vi "Main.vi"(8 "error in":errorcluster, 10 "Sequence Context":refnum<k7>, 11 "PostUUT":refnum<class "PostUUT.lvclass">) -> (0 "error out":errorcluster, 3 "PostUUT":refnum<class "PostUUT.lvclass">)   [LabVIEW 2019, in "Sequence Main.lvlib" / "PostUUT.lvclass"]
uses:
  PostUUT.lvclass
  C:/Workspace/gip-fct/Sequence/CodeModules/PreTestPost Launcher/Abstract UUT/Abstract UUT.lvclass
  PostUUT.lvclass/PostUUT.ctl
  Abstract UUT/Abstract UUT.lvclass
panel:
  out "MssgText":string
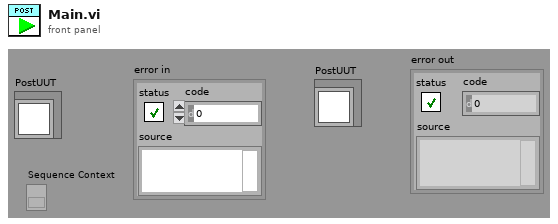
[diagram p1: front panel]
types:
  T1 = typedef "TestStand - Status Monitor.ctl" = cluster{"Sequence Context":refnum<k7>, "Execution":refnum<k7>, "Termination Monitor":refnum<k7>}
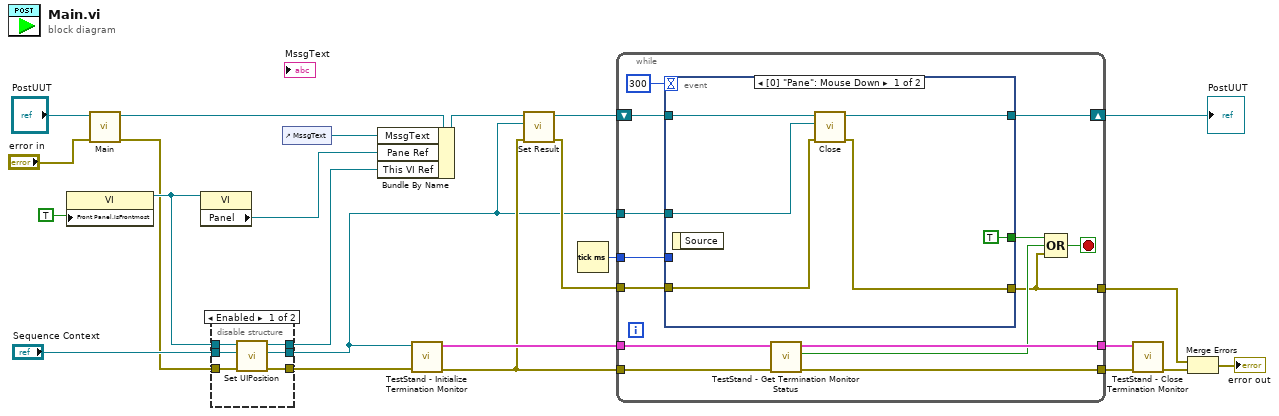
[diagram p0: block diagram]
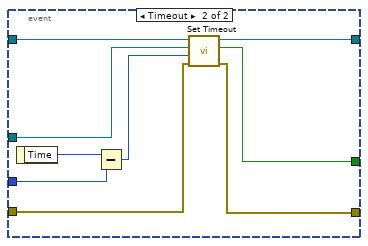
[diagram p3: hidden frame]
diagram:
  n1 = property class="VI"("Front Panel.IsFrontmost"=TRUE ("Front Panel Window:Is Frontmost")) -> (reference out=w15:refnum<vi>)  [unwired: 2 in, 1 out]
  n2 = call-parent "Main.vi"("error in"="error in", "OPC UA In"="PostUUT") -> ("error out"=w6:errorcluster, "OPC UA Out"=w7:refnum<class "PostUUT.lvclass">)  [unwired: 8 in]
  n3 = property class="VI"(reference=w15) -> ("Panel"=w23:refnum<vi>)  [unwired: 1 in, 2 out]
  n4 = disable-structure shown="Enabled" {
    disable-tunnel: [w30 w31] -> w17
    disable-tunnel: "Sequence Context" -> [w26 w32]
    disable-tunnel: w15 -> [w29 w33]
    disable-tunnel: [w28 w33] -> w14
    disable-tunnel: [w25 w32] -> w1
    disable-tunnel: w6 -> [w27 w31]
    frame Enabled {
      n5 = call "Set UIPosition.vi"("error in"=w27, "Sequence Context In"=w26, "VI Ref"=w29) -> ("error out"=w30:errorcluster, "Sequence Context out"=w25:refnum<k7>, "VI Ref out"=w28:refnum<vi>)  [unwired: 6 in]
    }
    frame Disabled {
    }
  }
  n6 = control-ref of="MssgText"() -> (w8:refnum<vi>)
  n7 = Bundle By Name(cluster=w7, "MssgText"=w8, "Pane Ref"=w23, "This VI Ref"=w14) -> (w5:refnum<class "PostUUT.lvclass">)
  n8 = call <vilib>:"TestStand - Initialize Termination Monitor.vi"("error in (no error)"=w17, "Sequence Context In"=w1) -> ("error out"=w3:errorcluster, "Status Monitor Out"=w22:T1)  [unwired: 8 in]
  n9 = call "Set Result.vi"("error in (no error)"=w3, "Sequence Context"=w1, "PostUUT in"=w5) -> ("error out"=w2:errorcluster, "PostUUT out"=w4:refnum<class "PostUUT.lvclass">)  [unwired: 7 in]
  n10 = Tick Count (ms)() -> (millisecond timer value=w11:u32)
  n11 = while {
    tunnel: w3 -> [w45]
    tunnel: w22 -> [w44]
    tunnel: [w38] -> w21
    tunnel: [w42] -> w20
    tunnel: w2 -> [w37]
    tunnel: [w36] -> w12
    tunnel: w11 -> [w35]
    shift-right: [w41] -> w9
    shift-left: w4 -> [w47]
    tunnel: w1 -> [w34]
    stop <- w43 stop-if-true
    n12 = event shown="[0] \"Pane\": Mouse Down" {
      selector: _ -> [_ _]
      dyn-events: _ -> [_ _]
      timeout: 300 -> [_ _]
      tunnel: w47 -> [w52 w60]
      tunnel: [w51 w59] -> w41
      tunnel: [TRUE ("Timeout") w56] -> w39
      tunnel: w37 -> [w50 w58]
      tunnel: [w49 w57] -> w36
      tunnel: w35 -> [_ w61]
      tunnel: w34 -> [w48 w54]
      event Mouse Down {
        n13 = event-data() -> ()  [unwired: 1 in, 1 out]
        n14 = call-dynamic "Close.vi"("error in (no error)"=w50, "Sequence Context"=w48, "PostUUT in"=w52) -> ("error out"=w49:errorcluster, "PostUUT out"=w51:refnum<class "PostUUT.lvclass">)  [unwired: 7 in]
      }
      event Timeout {
        n15 = event-data() -> ("Time"=w62:u32)  [unwired: 1 in]
        n16 = Subtract(x=w62, y=w61) -> (x-y=w55:u32)
        n17 = call "Set Timeout.vi"("error in (no error)"=w58, "Elapsed Time"=w55, "Sequence Context"=w54, "Abstract UUT in"=w60) -> ("error out"=w57:errorcluster, "Timeout"=w56:bool, "Abstract UUT out"=w59:refnum<class "PostUUT.lvclass">)  [unwired: 5 in]
      }
    }
    n18 = call <vilib>:"TestStand - Get Termination Monitor Status.vi"("error in (no error)"=w45, "Status Monitor In"=w44) -> ("error out"=w38:errorcluster, "Terminating or Aborting"=w40:bool, "Status Monitor Out"=w42:T1)  [unwired: 7 in]
    n19 = Compound Arithmetic op=OR(w39, w40, w36) -> (w43:bool)
  }
  "PostUUT" <- w9
  n20 = call <vilib>:"TestStand - Close Termination Monitor.vi"("error in (no error)"=w21, "Status Monitor In"=w20) -> ("error out"=w18:errorcluster)  [unwired: 9 in]
  n21 = Merge Errors(w12, w18) -> (→"error out":errorcluster)
